vi "Lakeshore 325 Set Control Parameters.vi"(8 "error in (no error)":errorcluster, 11 "Lakeshore 325 in":refnum<class "Lakeshore 325.lvclass">) -> (0 "error out":errorcluster, 3 "Lakeshore 325 out":refnum<class "Lakeshore 325.lvclass">)   [LabVIEW 2022 SP3, in "Lakeshore 325.lvclass"]
uses:
  Lakeshore 325.lvclass
  Lakeshore 325.lvclass/Lakeshore 325.ctl
  <instrlib>/Lake Shore 325/Lake Shore 325.lvlib
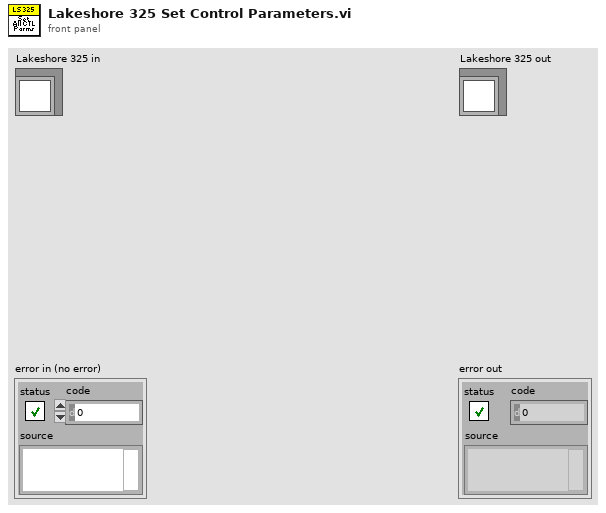
[diagram p1: front panel]
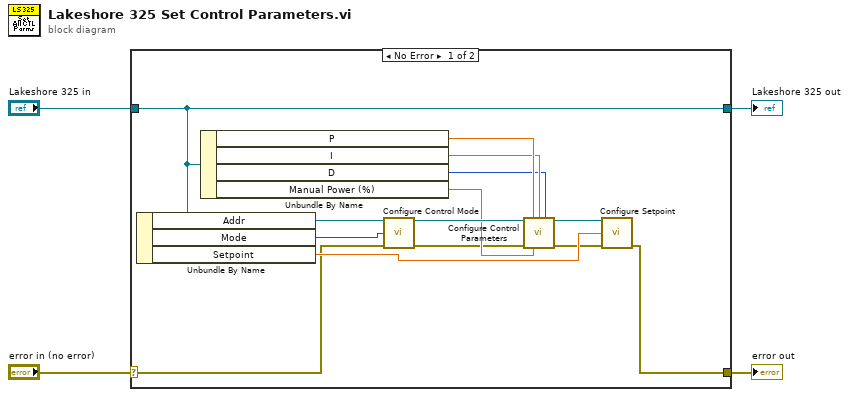
[diagram p0: block diagram]
diagram:
  n1 = case shown="No Error" "error in (no error)" {
    selector: "error in (no error)" -> [w5 w20]
    tunnel: [w6 w20] -> w3
    tunnel: [w15 w19] -> w1
    tunnel: "Lakeshore 325 in" -> [w15 w19]
    frame No Error {
      n2 = Unbundle By Name(w15) -> ("Addr"=w18:refnum<visa-resource-name>, "Mode"=w17:u16, "Setpoint"=w8:dbl)
      n3 = Unbundle By Name(w15) -> ("P"=w14:dbl, "I"=w13:dbl, "D"=w12:u16, "Manual Power (%)"=w11:dbl)
      n4 = call <instrlib>:"Configure Control Mode.vi"("VISA resource name"=w18, "Mode (1:Manual PID)"=w17, "error in (no error)"=w5) -> ("VISA resource name out"=w16:refnum<visa-resource-name>, "error out"=w10:errorcluster)  [unwired: 11 in]
      n5 = call <instrlib>:"Configure Control Parameters.vi"("VISA resource name"=w16, "Gain (P) (0.0)"=w14, "Reset (I) (0.0)"=w13, "Rate (D) (0 %)"=w12, "error in (no error)"=w10, "Manual Heater Power (0.000 %)"=w11) -> ("VISA resource name out"=w9:refnum<visa-resource-name>, "error out"=w7:errorcluster)  [unwired: 8 in]
      n6 = call <instrlib>:"Configure Setpoint.vi"("VISA resource name"=w9, "Setpoint Value (0.0000)"=w8, "error in (no error)"=w7) -> ("error out"=w6:errorcluster)  [unwired: 11 in, 1 out]
    }
    frame Error {
    }
  }
  "error out" <- w3
  "Lakeshore 325 out" <- w1
